vi "Direction Cosines To Euler Angles.vi"(10 "rotation order":T1=10 items=["X-Y-Z", "X-Z-Y", "Y-X-Z", "Y-Z-X", "Z-X-Y", "Z-Y-X", "X-Y-X", "X-Z-X", "Y-X-Y", "Y-Z-Y", "Z-X-Z", "Z-Y-Z"], 11 "Direction Cosines":dbl[][](array[numeric])) -> (0 "error":i32, 3 "Euler Angles":cluster{"phi":dbl, "theta":dbl, "psi":dbl})   [LabVIEW 2024, in "NI_AALPro.lvlib"]
doc: "<p>Converts a 3-by-3 matrix of direction cosines into Euler angles.</p>"
uses:
  NI_AALPro.lvlib
  Euler Rotation Order.ctl
  <resource>/lvanlys.dll
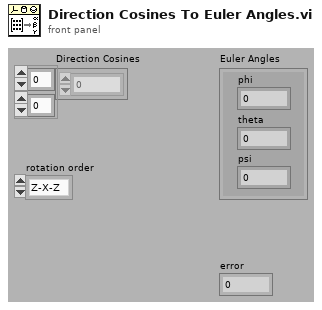
[diagram p1: front panel]
types:
  T1 = typedef "NI_AALPro.lvlib/Euler Rotation Order.ctl" = u16
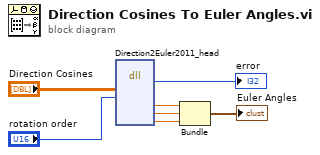
[diagram p0: block diagram]
diagram:
  n1 = dll-call lib="C:/Program Files (x86)/National Instruments/LabVIEW 2024/resource/lvanlys.*" fn="Direction2Euler2011_head"("direction"="Direction Cosines", "rotateOrder"="rotation order") -> ("return type"=→"error":i32, "phi"=w5:dbl, "theta"=w4:dbl, "psi"=w3:dbl)  [unwired: 8 in, 2 out]
  n2 = Bundle("phi"=w5, "theta"=w4, "psi"=w3) -> (→"Euler Angles":cluster{"phi":dbl, "theta":dbl, "psi":dbl})  [unwired: 1 in]
